vi "fast_cmd_compose.vi"(0 "Input Double (0.0)":dbl, 4 "Input I32 (0)":i32, 5 "*WAI (F)":bool, 6 "Input I64 (0)":i64, 7 "Data Type in":i32, 8 "Input Boolean (F)":bool, 9 "Input String (\"\")":string, 10 "Direct cmd in":string, 11 "SCPI Command without parameter":string) -> (2 "Direct cmd out":string, 3 "Complete SCPI Command":string)   [LabVIEW 2014, in "rszvl_rsidr_core.lvlib"]
uses:
  rszvl_rsidr_core.lvlib
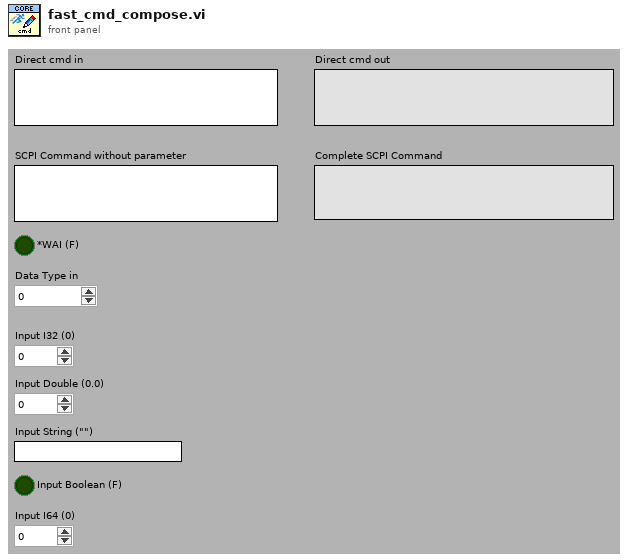
[diagram p1: front panel]
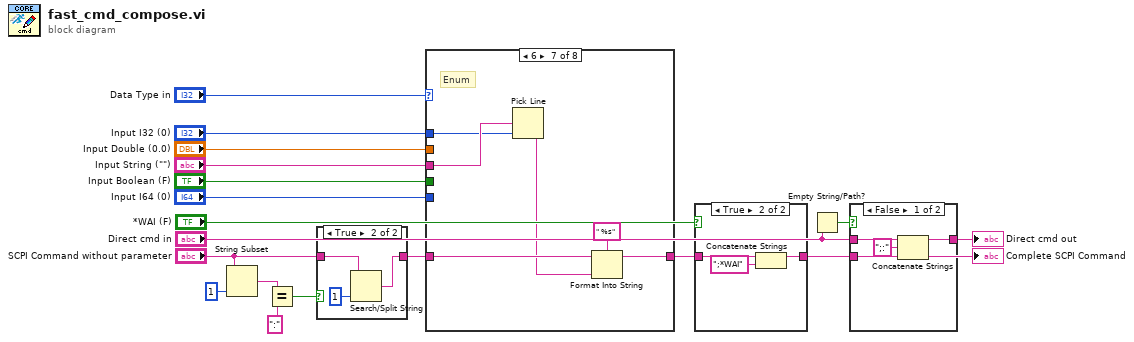
[diagram p0: block diagram]
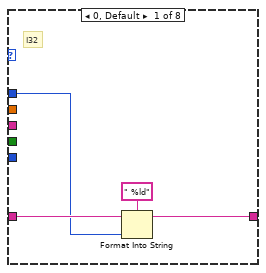
[diagram p5: hidden frame]
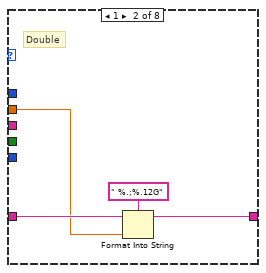
[diagram p6: hidden frame]
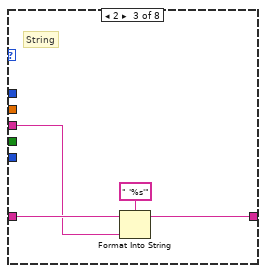
[diagram p7: hidden frame]
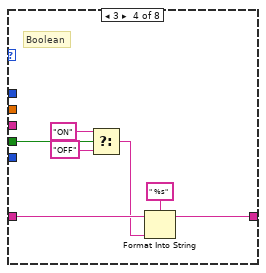
[diagram p8: hidden frame]
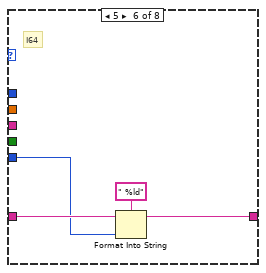
[diagram p10: hidden frame]
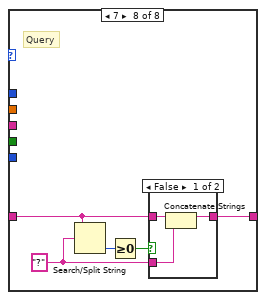
[diagram p11: hidden frame]
diagram:
  n1 = String Subset(string="SCPI Command without parameter", length (rest)=1 ("length (rest)")) -> (substring=w6:string)  [unwired: 1 in]
  n2 = Equal?(x=w6, y=":" ("search string/char (-)")) -> (x = y?=w4:bool)
  n3 = case shown="True" w4 {
    tunnel: "SCPI Command without parameter" -> [w19 w22]
    tunnel: [w19 w20] -> w12
    frame False {
    }
    frame True {
      n4 = Search/Split String(string=w22, offset (0)=1) -> (match + rest of string=w20:string)  [unwired: 1 in, 2 out]
    }
  }
  n5 = case shown="6" "Data Type in" {
    tunnel: "Input I32 (0)" -> [w24 _ _ _ _ _ w47 _]
    tunnel: w12 -> [w25 w29 w33 w40 w42 w45 w51 w55]
    tunnel: [w23 w28 w32 w39 w42 w44 w50 w54] -> w2
    tunnel: "Input Double (0.0)" -> [_ w27 _ _ _ _ _ _]
    tunnel: "Input String (\"\")" -> [_ _ w31 _ _ _ w49 _]
    tunnel: "Input Boolean (F)" -> [_ _ _ w36 _ _ _ _]
    tunnel: "Input I64 (0)" -> [_ _ _ _ _ w43 _ _]
    frame 0, Default {
      # "I32"
      n6 = Format Into String(format string=" %ld", initial string=w25, w24) -> (resulting string=w23:string)  [unwired: 1 in, 1 out]
    }
    frame 1 {
      # "Double"
      n7 = Format Into String(format string=" %.;%.12G", initial string=w29, w27) -> (resulting string=w28:string)  [unwired: 1 in, 1 out]
    }
    frame 2 {
      # "String"
      n8 = Format Into String(format string=" '%s'", initial string=w33, w31) -> (resulting string=w32:string)  [unwired: 1 in, 1 out]
    }
    frame 3 {
      # "Boolean"
      n9 = Select(t="ON", s=w36, f="OFF") -> (s? t:f=w35:string)
      n10 = Format Into String(format string=" %s", initial string=w40, w35) -> (resulting string=w39:string)  [unwired: 1 in, 1 out]
    }
    frame 4 {
      # "Event"
    }
    frame 5 {
      # "I64"
      n11 = Format Into String(format string=" %ld", initial string=w45, w43) -> (resulting string=w44:string)  [unwired: 1 in, 1 out]
    }
    frame 6 {
      # "Enum"
      n12 = Pick Line(multi-line string=w49, line index=w47) -> (output string=w48:string)  [unwired: 1 in]
      n13 = Format Into String(format string=" %s", initial string=w51, w48) -> (resulting string=w50:string)  [unwired: 1 in, 1 out]
    }
    frame 7 {
      w57 = "?" ("search string/char (-)")
      # "Query"
      n14 = Search/Split String(string=w55, search string/char (-)=w57) -> (offset of match=w56:i32)  [unwired: 1 in, 2 out]
      n15 = Greater Or Equal To 0?(x=w56) -> (x >= 0?=w53:bool)
      n16 = case shown="False" w53 {
        tunnel: w57 -> [w59 _]
        tunnel: w55 -> [w60 w61]
        tunnel: [w58 w61] -> w54
        frame False {
          n17 = Concatenate Strings(w60, w59) -> (w58:string)
        }
        frame True {
        }
      }
    }
  }
  n18 = case shown="True" "*WAI (F)" {
    tunnel: w2 -> [w62 w65]
    tunnel: [w62 w64] -> w1
    frame False {
    }
    frame True {
      n19 = Concatenate Strings(w65, ";*WAI" ("string")) -> (w64:string)
    }
  }
  "Complete SCPI Command" <- w1
  n20 = Empty String/Path?(string/path="Direct cmd in") -> (empty?=w11:bool)
  n21 = case shown="False" w11 {
    tunnel: w1 -> [w67 w70]
    tunnel: "Direct cmd in" -> [w69 _]
    tunnel: [w66 w70] -> w9
    frame False {
      n22 = Concatenate Strings(w69, ";:" ("string"), w67) -> (w66:string)
    }
    frame True {
    }
  }
  "Direct cmd out" <- w9
